vi "convertADCstring.vi"(11 "String":string) -> ()   [LabVIEW 2014]
uses:
  controls/Graph Data.ctl
  <vilib>/Utility/miscctls.llb/LVAnnotationListTypeDef.ctl
  <vilib>/Utility/miscctls.llb/LVCursorListTypeDef.ctl
panel:
  in  "Enum":enum16{"ADC16", "ADC18"}(ring)
  out "Array - Numeric 11":dbl[](array[numeric])
  out "Array - Numeric":dbl[](array[numeric])
  out "Channel 8":dbl[](array[numeric])
  out "Channel 7":dbl[](array[numeric])
  out "Channel 6":dbl[](array[numeric])
  out "Channel 5":dbl[](array[numeric])
  out "Channel 4":dbl[](array[numeric])
  out "Channel 3":dbl[](array[numeric])
  out "Channel 2":dbl[](array[numeric])
  out "Channel 1":dbl[](array[numeric])
  out "Numeric 2":dbl
  out "Array - String":string[](array[string])
  in  "Graph Data":T1
  out "Numeric":i32
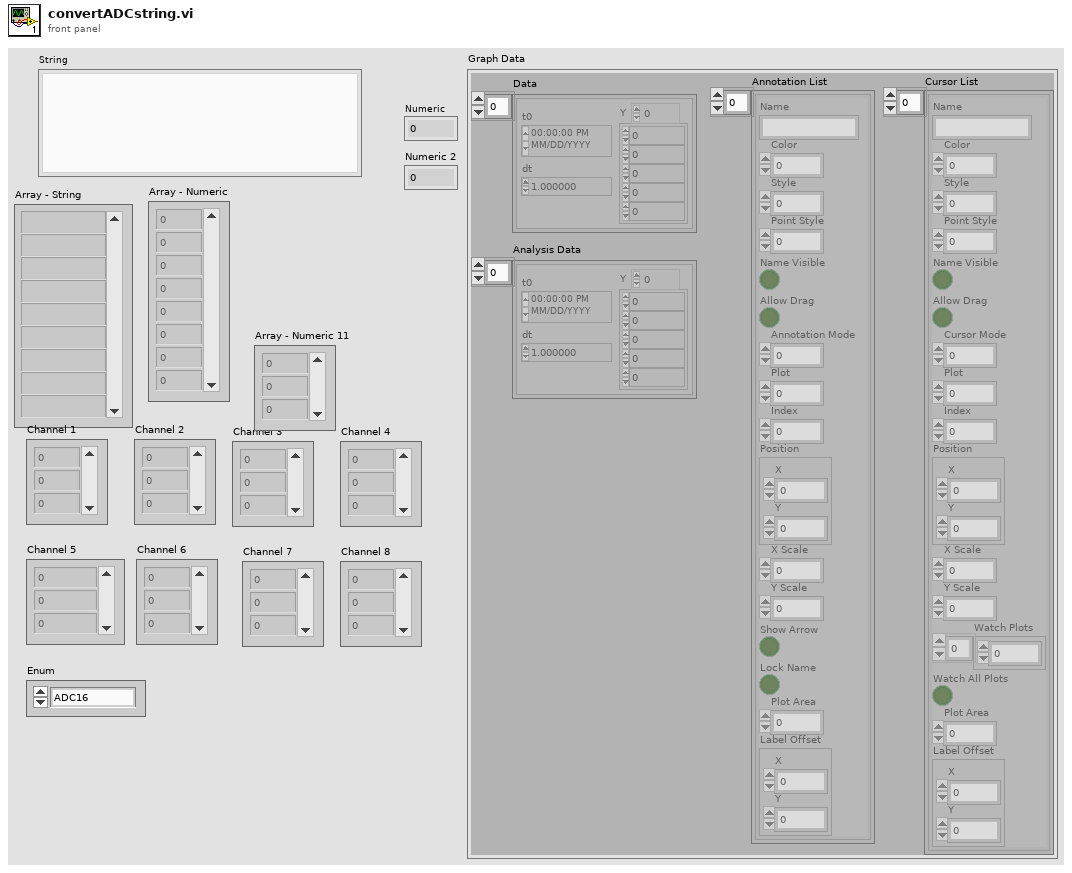
[diagram p1: front panel]
types:
  T1 = typedef "Graph Data.ctl" = cluster{"Data":waveform(dbl)[], "Annotation List":T2, "Cursor List":T3, "Analysis Data":waveform(dbl)[]}
  T2 = typedef "LVAnnotationListTypeDef.ctl" = cluster{"Name":string, "Color":u32, "Style":u8, "Point Style":u8, "Name Visible":bool, "Allow Drag":bool, "Annotation Mode":u32, "Plot":i32, "Index":i32, "Position":cluster{"X":dbl, "Y":dbl}, "X Scale":u32, "Y Scale":u32, "Show Arrow":bool, "Lock Name":bool, "Plot Area":i32, "Label Offset":cluster{"X":dbl, "Y":dbl}}[]
  T3 = typedef "LVCursorListTypeDef.ctl" = cluster{"Name":string, "Color":u32, "Style":u8, "Point Style":u8, "Name Visible":bool, "Allow Drag":bool, "Cursor Mode":u32, "Plot":i32, "Index":i32, "Position":cluster{"X":dbl, "Y":dbl}, "X Scale":u32, "Y Scale":u32, "Watch Plots":i32[], "Watch All Plots":bool, "Plot Area":i32, "Label Offset":cluster{"X":dbl, "Y":dbl}}[]
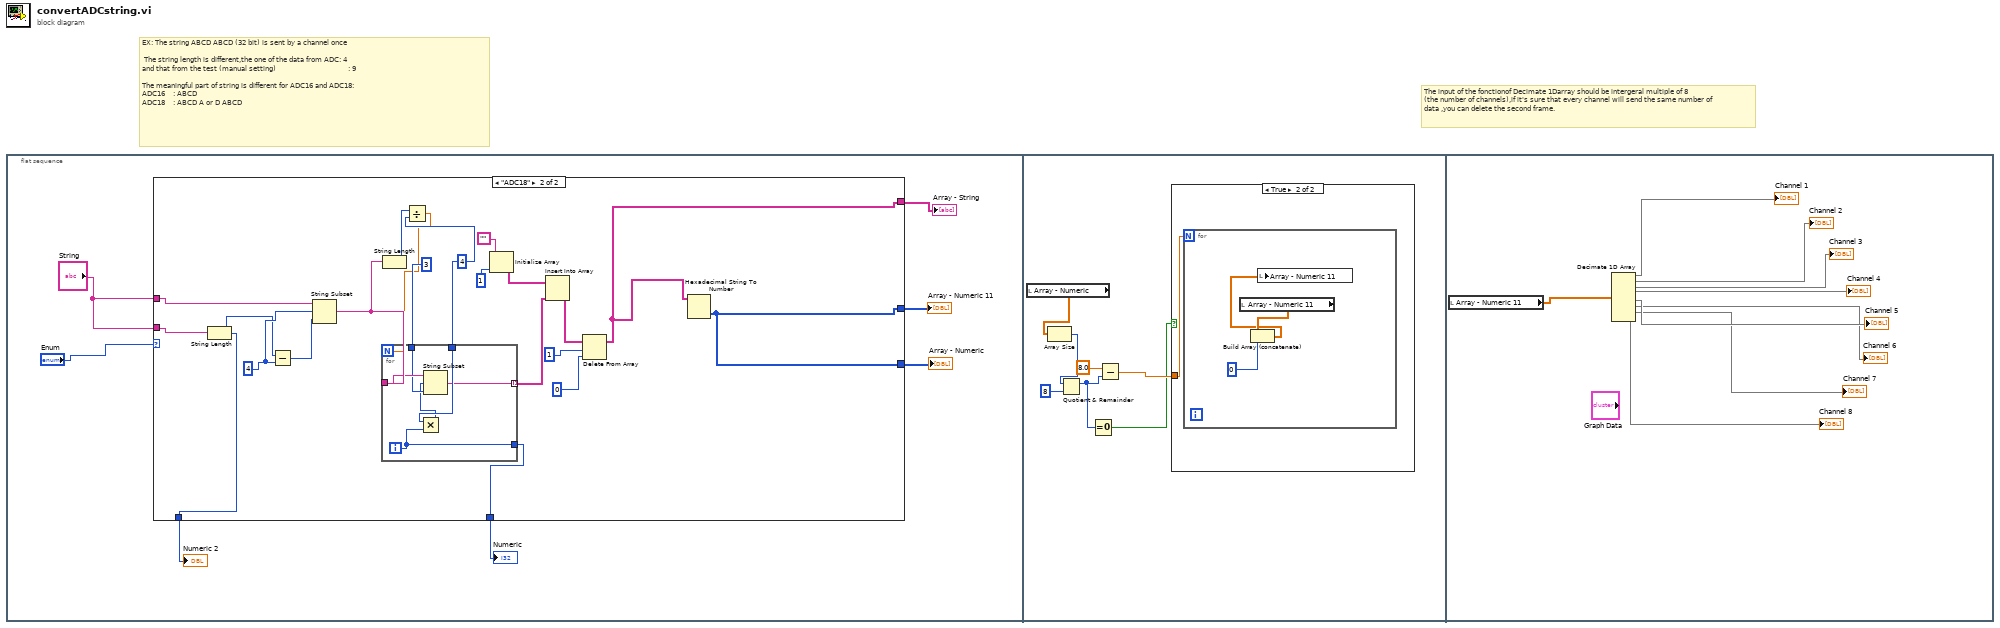
[diagram p0: block diagram]
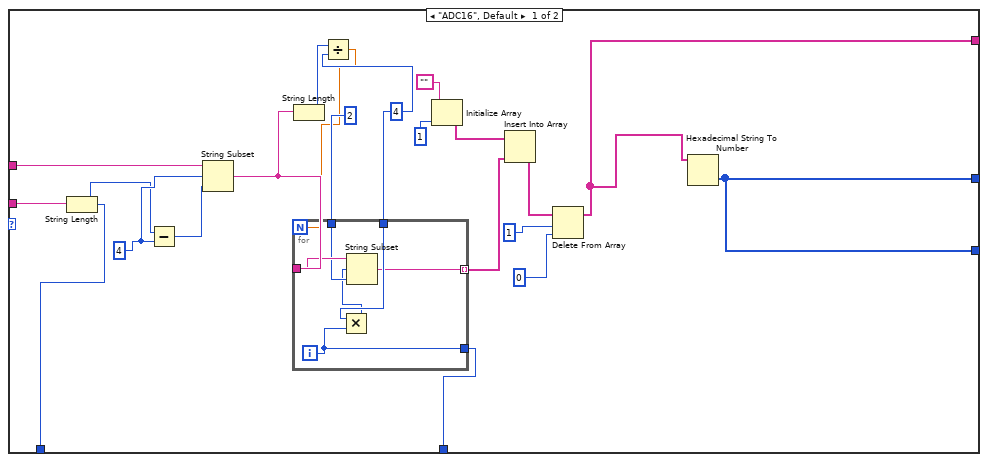
[diagram p2: hidden frame]
diagram:
  # "The input of the fonctionof Decimate 1Darray should be intergeral multiple of 8\n(the number of channels),if it's sure that every channel will send the same number of data ,you can delete the second frame."
  # "EX: The string ABCD ABCD (32 bit) is sent by a channel once                \n\n The string length is different,the one of the data from ADC: 4\nand that from the test (manual setting)                                    : 9\n\nThe meaningful part of string is different for ADC16 and ADC18:\nADC16    : ABCD                          \nADC18    : ABCD A or D ABCD"
  n1 = flat-sequence {
    frame #0 {
      n2 = case shown="\"ADC18\"" "Enum" {
        tunnel: "String" -> [w13 w39]
        tunnel: "String" -> [w12 w38]
        tunnel: [w11 w37] -> w6
        tunnel: [w11 w37] -> w5
        tunnel: [w10 w36] -> w4
        tunnel: [w9 w35] -> w3
        tunnel: [w8 w34] -> w2
        frame "ADC16", Default {
          w22 = 4
          w26 = 4
          n3 = String Length(string=w13) -> (length=w10:i32)
          n4 = Subtract(x=w10, y=w26) -> (x-y=w27:i32)
          n5 = String Subset(string=w12, offset (0)=w26, length (rest)=w27) -> (substring=w25:string)
          n6 = String Length(string=w25) -> (length=w23:i32)
          n7 = Divide(x=w23, y=w22) -> (x/y=w21:dbl)
          n8 = for {
            N: w21 -> [_]
            tunnel: w25 -> [w33]
            tunnel: 2 -> [w32]
            tunnel: w22 -> [w31]
            tunnel: [w29] -> w9
            tunnel: [w28] -> w14 mode=indexing
            i -> [w29]
            n9 = Multiply(x=w31, y=w29) -> (x*y=w30:i32)
            n10 = String Subset(string=w33, offset (0)=w30, length (rest)=w32) -> (substring=w28:string)
          }
          n11 = Initialize Array("", 1) -> (w18:string[])
          n12 = Insert Into Array(array=w18, new element=w14) -> (w17:string[])  [unwired: 1 in]
          n13 = Delete From Array(array=w17, length=1, index=0) -> (array with subset deleted=w8:string[])  [unwired: 1 out]
          n14 = Hexadecimal String To Number(string=w8) -> (number=w11:u32[])  [unwired: 2 in, 1 out]
        }
        frame "ADC18" {
          w48 = 4
          w52 = 4
          n15 = String Length(string=w39) -> (length=w36:i32)
          n16 = Subtract(x=w36, y=w52) -> (x-y=w53:i32)
          n17 = String Subset(string=w38, offset (0)=w52, length (rest)=w53) -> (substring=w51:string)
          n18 = String Length(string=w51) -> (length=w49:i32)
          n19 = Divide(x=w49, y=w48) -> (x/y=w47:dbl)
          n20 = for {
            N: w47 -> [_]
            tunnel: w51 -> [w59]
            tunnel: 3 -> [w58]
            tunnel: w48 -> [w57]
            tunnel: [w55] -> w35
            tunnel: [w54] -> w40 mode=indexing
            i -> [w55]
            n21 = Multiply(x=w57, y=w55) -> (x*y=w56:i32)
            n22 = String Subset(string=w59, offset (0)=w56, length (rest)=w58) -> (substring=w54:string)
          }
          n23 = Initialize Array("", 1) -> (w44:string[])
          n24 = Insert Into Array(array=w44, new element=w40) -> (w43:string[])  [unwired: 1 in]
          n25 = Delete From Array(array=w43, length=1, index=0) -> (array with subset deleted=w34:string[])  [unwired: 1 out]
          n26 = Hexadecimal String To Number(string=w34) -> (number=w37:u32[])  [unwired: 2 in, 1 out]
        }
      }
      "Array - Numeric 11" <- w5
      "Array - Numeric" <- w6
      "Numeric 2" <- w4
      "Numeric" <- w3
      "Array - String" <- w2
    }
    frame #1 {
      n27 = local read "Array - Numeric"() -> (w66:dbl[])
      n28 = Array Size(array=w66) -> (size(s)=w64:i32)
      n29 = Quotient & Remainder(x=w64, y=8) -> (x-y*floor(x/y)=w61:i32)  [unwired: 1 out]
      n30 = Equal To 0?(x=w61) -> (x = 0?=w60:bool)
      n31 = Subtract(x=8.0, y=w61) -> (x-y=w62:dbl)
      n32 = case shown="True" w60 {
        tunnel: w62 -> [_ w67]
        frame False {
        }
        frame True {
          n33 = for {
            N: w67 -> [_]
            n34 = local read "Array - Numeric 11"() -> (w69:dbl[])
            n35 = Build Array (concatenate)(w69, 0) -> (w68:dbl[])
            n36 = local write "Array - Numeric 11"(w68) -> ()
          }
        }
      }
    }
    frame #2 {
      n37 = local read "Array - Numeric 11"() -> (w71:dbl[])
      n38 = Decimate 1D Array(w71) -> (→"Channel 1":dbl[], →"Channel 2":dbl[], →"Channel 3":dbl[], →"Channel 4":dbl[], →"Channel 5":dbl[], →"Channel 6":dbl[], →"Channel 7":dbl[], →"Channel 8":dbl[])
    }
  }
